vi "is abstract.vi"(8 "error in":errorcluster, 11 "NISE_CEF_serializable node in":refnum<class "NISE_CEF_serializable node.lvclass">) -> (0 "error out":errorcluster, 2 "abstract":bool, 3 "NISE_CEF_serializable node out":refnum<class "NISE_CEF_serializable node.lvclass">)   [LabVIEW 2013, in "NISE_CEF_serializable node.lvclass"]
uses:
  NISE_CEF_serializable node.lvclass
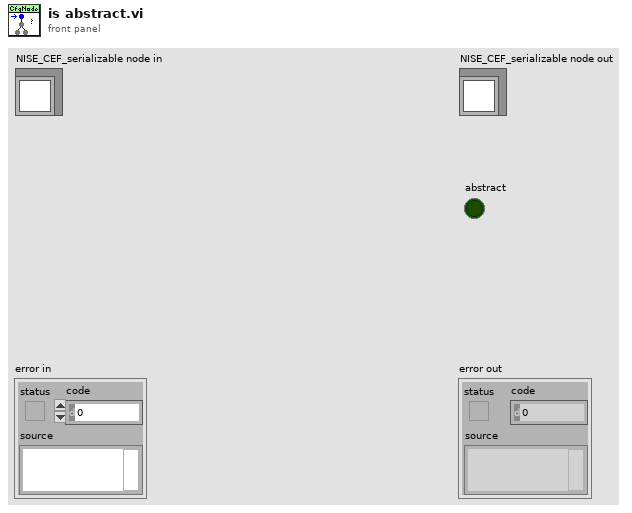
[diagram p1: front panel]
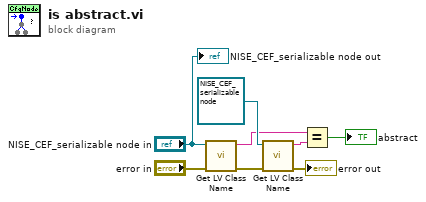
[diagram p0: block diagram]
diagram:
  n1 = call <vilib>:"Get LV Class Name.vi"("error in (no error)"="error in", "object"="NISE_CEF_serializable node in") -> ("error out"=w6:errorcluster, "class name"=w4:string)  [unwired: 8 in]
  n2 = call <vilib>:"Get LV Class Name.vi"("error in (no error)"=w6, "object"=refnum<class "NISE_CEF_serializable node.lvclass"> refnum ("NISE_CEF_serializable node.lvclass")) -> ("error out"=→"error out":errorcluster, "class name"=w5:string)  [unwired: 8 in]
  n3 = Equal?(x=w4, y=w5) -> (x = y?=→"abstract":bool)
  "NISE_CEF_serializable node out" <- "NISE_CEF_serializable node in"
